vi "LakeShore370 Get Controls.vi"(8 "error in (no error)":errorcluster, 10 "Control Panel Data":T1={"Channels to scan"=[], "Scan settling, s"=10.0, "Read temperature"=FALSE, "Set point"=0.0, "Heater range"=enum."Off", "Approach"=enum."Instant", "Ramp rate, K/min"=1.0, "Read heater"=FALSE}, 11 "VISA resource name":refnum<visa-resource-name>) -> (0 "error out":errorcluster, 2 "Control Panel Data Out":T1={"Channels to scan"=[], "Scan settling, s"=10.0, "Read temperature"=FALSE, "Set point"=0.0, "Heater range"=enum."Off", "Approach"=enum."Instant", "Ramp rate, K/min"=1.0, "Read heater"=FALSE}, 3 "VISA Resource Name Out":refnum<visa-resource-name>)   [LabVIEW 2015]
uses:
  LakeSore370 Front Panel Data.ctl
  LakeShore370 Heater Ranges.ctl
  Neocera/Neocera Set Point Aproach.ctl
  GPIB/VISA  Send Receive.vi
panel:
  out "data string out":string
  out "data string":string
  # "Scanner"
  # "Temperature Control"
  # "Scanner"
  # "Temperature Control"
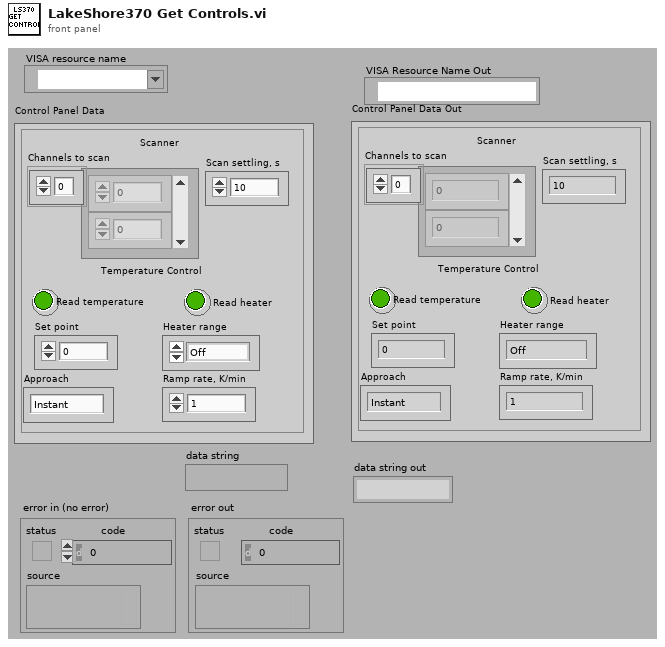
[diagram p1: front panel]
types:
  T1 = typedef "LakeSore370 Front Panel Data.ctl" = cluster{"Channels to scan":i32[], "Scan settling, s":dbl, "Read temperature":bool, "Set point":dbl, "Heater range":T2, "Approach":T3, "Ramp rate, K/min":dbl, "Read heater":bool}
  T2 = typedef "LakeShore370 Heater Ranges.ctl" = enum16{"Off", "31.6uA", "100uA", "316uA", "1mA", "3.16uA", "10mA", "31.6mA", "100mA"}
  T3 = typedef "Neocera Set Point Aproach.ctl" = enum16{"Instant", "Ramp"}
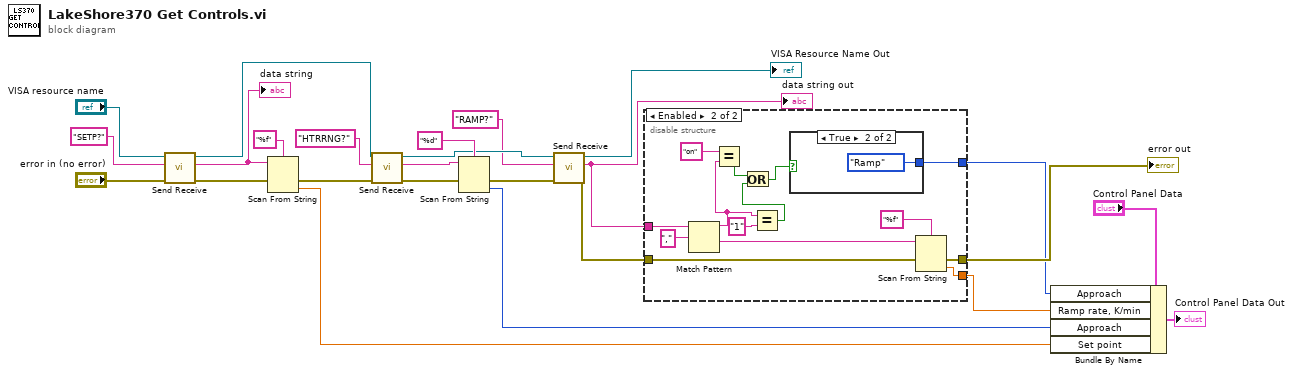
[diagram p0: block diagram]
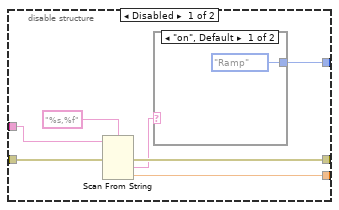
[diagram p2: hidden frame]
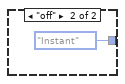
[diagram p3: hidden frame]
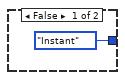
[diagram p4: hidden frame]
diagram:
  n1 = call-poly "Send Receive.vi"("error in (no error)"="error in (no error)", "data string in"="SETP?" ("data string"), "VISA Resource Name"="VISA resource name") -> ("error out"=w22:errorcluster, "data string out"=w18:string, "VISA Resource Name Out"=w11:refnum<visa-resource-name>)  [unwired: 6 in]
  "data string" <- w18
  n2 = Scan From String(format string="%f", input string=w18, error in=w22) -> (error out=w15:errorcluster, output 1=w2:dbl)  [unwired: 2 in, 2 out]
  n3 = call-poly "Send Receive.vi"("error in (no error)"=w15, "data string in"="HTRRNG?", "VISA Resource Name"=w11) -> ("error out"=w14:errorcluster, "data string out"=w13:string, "VISA Resource Name Out"=w12:refnum<visa-resource-name>)  [unwired: 6 in]
  n4 = Scan From String(format string="%d", input string=w13, error in=w14) -> (error out=w4:errorcluster, output 1=w3:i32)  [unwired: 2 in, 2 out]
  n5 = call-poly "Send Receive.vi"("error in (no error)"=w4, "data string in"="RAMP?" ("format string"), "VISA Resource Name"=w12) -> ("error out"=w17:errorcluster, "data string out"=w1:string, "VISA Resource Name Out"=→"VISA Resource Name Out":refnum<visa-resource-name>)  [unwired: 6 in]
  "data string out" <- w1
  n6 = disable-structure shown="Enabled" {
    disable-tunnel: w17 -> [w32 w44]
    disable-tunnel: [w31 w43] -> w10
    disable-tunnel: [w29 w48] -> w7
    disable-tunnel: [w28 w41] -> w6
    disable-tunnel: w1 -> [w27 w47]
    frame Disabled {
      n7 = Scan From String(format string="%s,%f", input string=w27, error in=w32) -> (error out=w31:errorcluster, output 1=w30:string, output 2=w28:dbl)  [unwired: 3 in, 2 out]
      n8 = case shown="\"on\", Default" w30 {
        tunnel: [Neocera_Set_Point_Aproach."Ramp" ("Approach") Neocera_Set_Point_Aproach."Instant" ("Approach")] -> w29
        frame "on", Default {
        }
        frame "off" {
        }
      }
    }
    frame Enabled {
      n9 = Match Pattern(string=w47, regular expression=",") -> (before substring=w37:string, after substring=w42:string)  [unwired: 1 in, 2 out]
      n10 = Equal?(x="on", y=w37) -> (x = y?=w35:bool)
      n11 = Equal?(x=w37, y="1" ("x")) -> (x = y?=w39:bool)
      n12 = Or(x=w35, y=w39) -> (x .or. y?=w38:bool)
      n13 = case shown="True" w38 {
        tunnel: [Neocera_Set_Point_Aproach."Instant" ("Approach") Neocera_Set_Point_Aproach."Ramp" ("Approach")] -> w48
        frame False {
        }
        frame True {
        }
      }
      n14 = Scan From String(format string="%f", input string=w42, error in=w44) -> (error out=w43:errorcluster, output 1=w41:dbl)  [unwired: 2 in, 2 out]
    }
  }
  "error out" <- w10
  n15 = Bundle By Name(cluster="Control Panel Data", "Approach"=w7, "Ramp rate, K/min"=w6, "Approach"=w3, "Set point"=w2) -> (→"Control Panel Data Out":T1)
